vi "WaveGraphView.vi"() -> ()   [LabVIEW 2014]
uses:
  GlobalData/GlobalData.vi
panel:
  in  "btnInitial":bool
  in  "太線(+3)":bool
  in  "自動スケール":bool
  in  "軸本数":u16(ring)=4 items=["２"=2, "４"=4, "６"=6, "８"=8]
  in  "MIN":dbl format="%#_6f"
  in  "MAX":dbl format="%#_6f"
  in  "Y軸":u16(ring) items=["No.", "時間HH:MM:SS.S", "M1回転rpm", "M2回転rpm", "M3回転rpm", "M1トルクN･m", "M2トルクN･m", "M3トルクN･m"]
  in  "プロットCH":u16(ring) items=["No.", "時間HH:MM:SS.S", "M1回転rpm", "M2回転rpm", "M3回転rpm", "M1トルクN･m", "M2トルクN･m", "M3トルクN･m", "", "", "", "", "", "", "", "", "", "", "供試体温度1℃", "供試体温度2℃", "供試体温度3℃", "動力盤温度℃", "軸受温度1℃", "軸受温度2℃", "軸受温度3℃", "", "効率"]
  in  "名称":string
  in  "色":u32(colorbox)
  in  "btnAddCursor":bool
  in  "btnScaleLegendVis":bool
  in  "btnLegVis":bool
  in  "btnCursorLegendVis":bool
  out "波形グラフ":waveform(dbl)[](graph)
  # "表示"
  # "カーソル"
  # "グラフCH設定"
  # "右クリック→カーソルを作成→複数プロット。さらに右クリック→監視→全てのプロット"
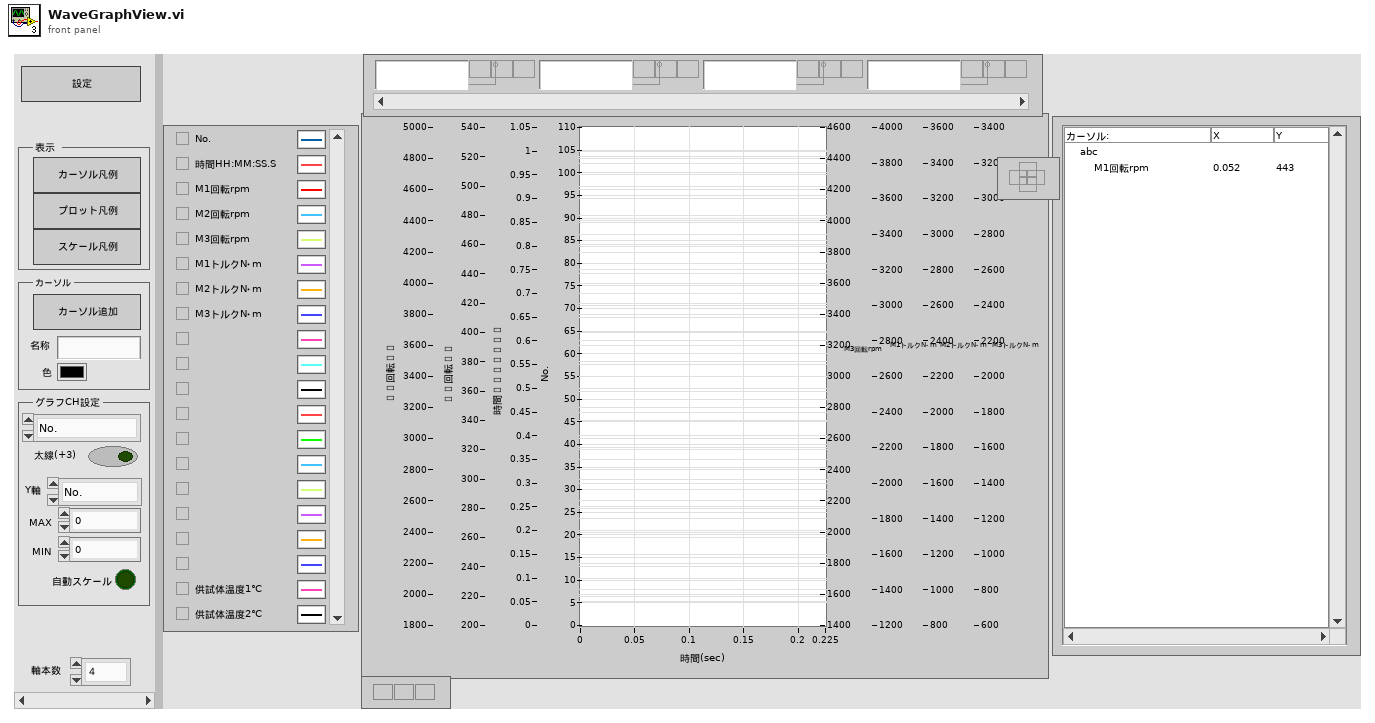
[diagram p1: front panel]
types:
  T1 = typedef "eventvkey.ctl" = enum16{"ASCII", "Enter", "Return", "Shift", "Ctrl", "Alt", "Cmd", "Opt", "Caps", "NumLock", "Clear", "Break", "Up", "Down", "Left", "Right", "Insert", "Delete", "Home", "End", "PageUp", "PageDown", "Escape", "Help", "Pause", "ScrollLock", "F1", "F2", "F3", "F4", "F5", "F6", "F7", "F8", "F9", "F10", "F11", "F12", "F13", "F14", "F15", "F16", "F17", "F18", "F19", "F20", "F21", "F22", "F23", "F24", "Play", "VolumeUp", "VolumeDown", "Mute", "Two Byte Char"}
  T2 = typedef "LVRangeTypeDef.ctl" = cluster{"Minimum":dbl, "Maximum":dbl, "Increment":dbl, "Minor Increment":dbl, "Start":dbl}
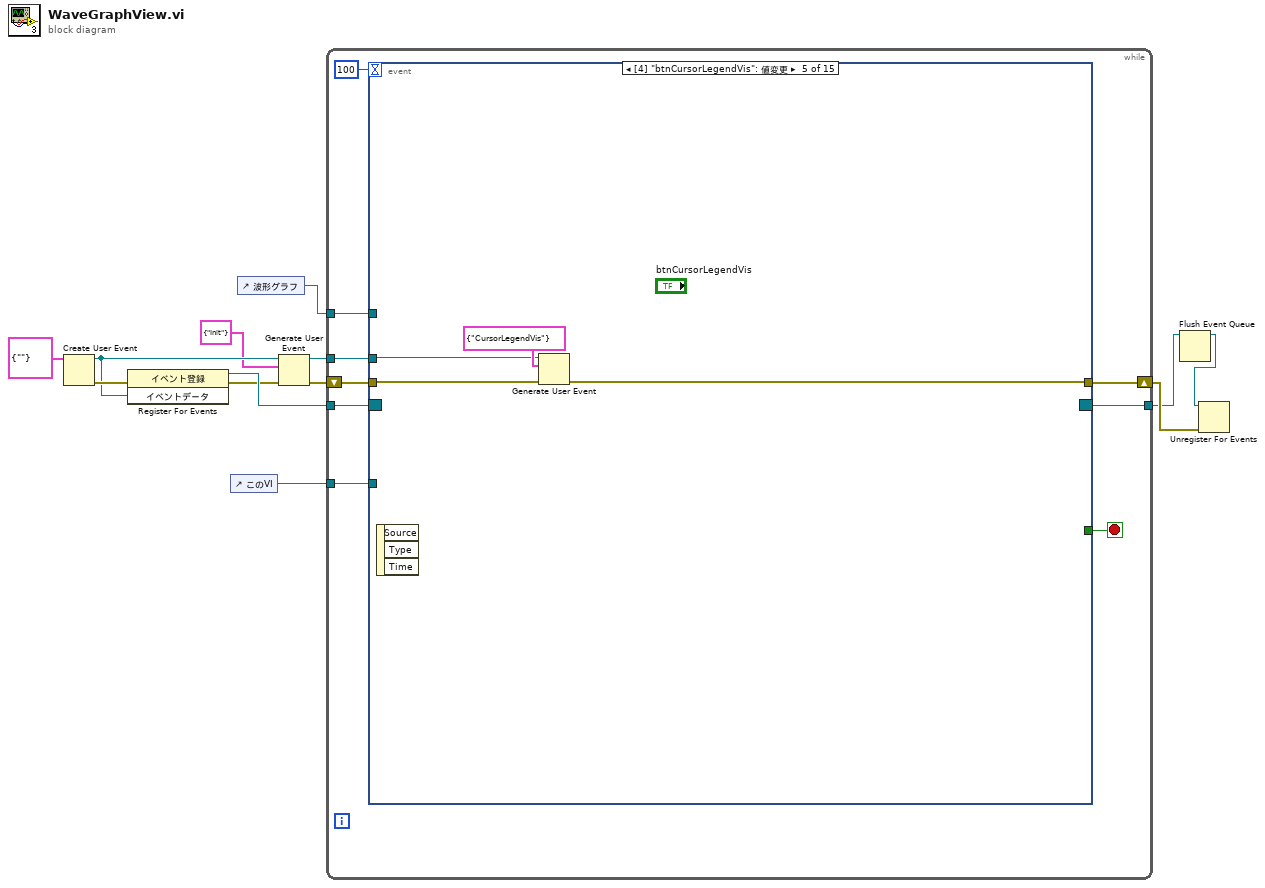
[diagram p0: block diagram]
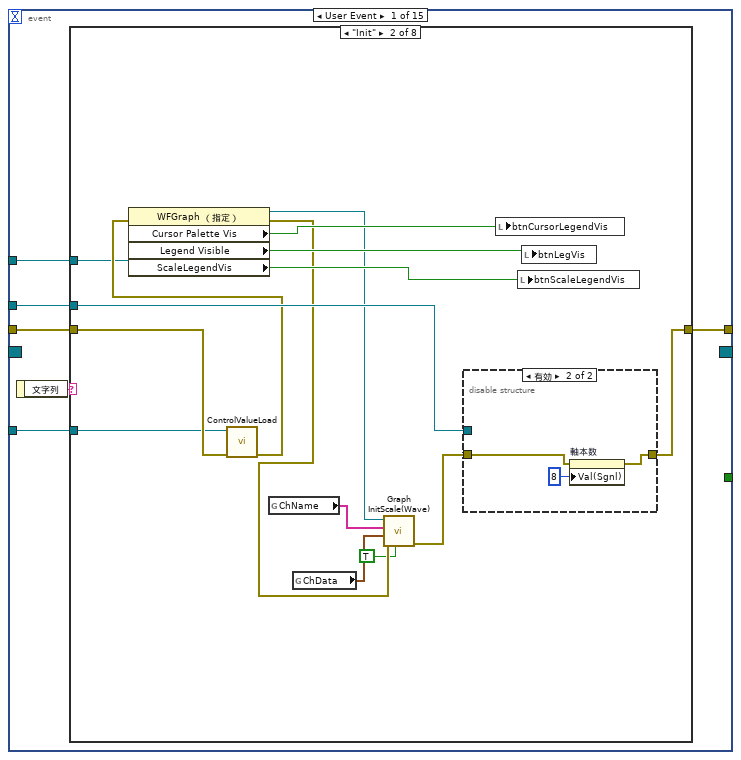
[diagram p2: hidden frame]
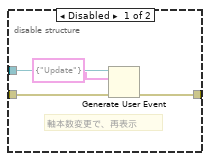
[diagram p4: hidden frame]
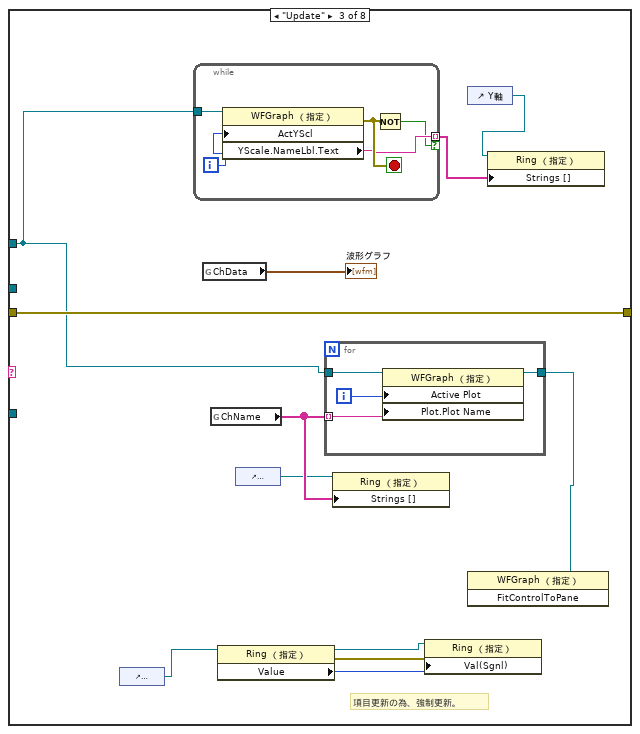
[diagram p5: hidden frame]
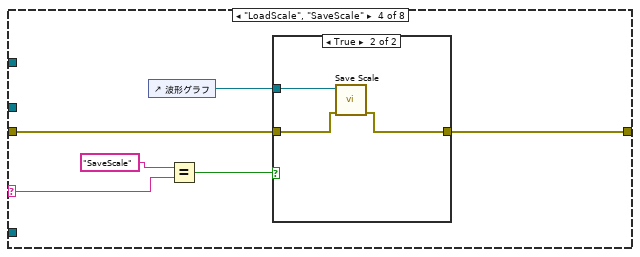
[diagram p6: hidden frame]
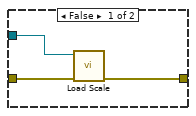
[diagram p7: hidden frame]
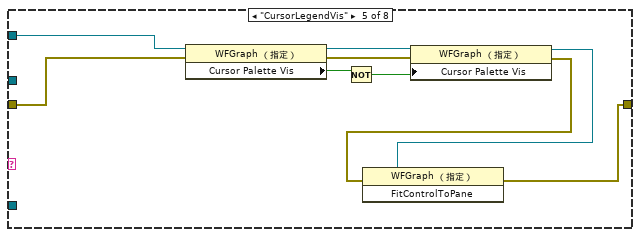
[diagram p8: hidden frame]
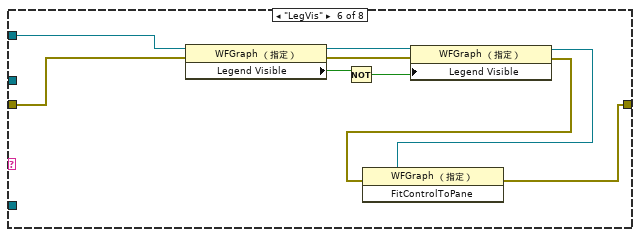
[diagram p9: hidden frame]
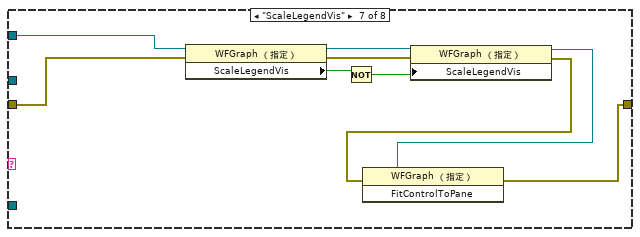
[diagram p10: hidden frame]
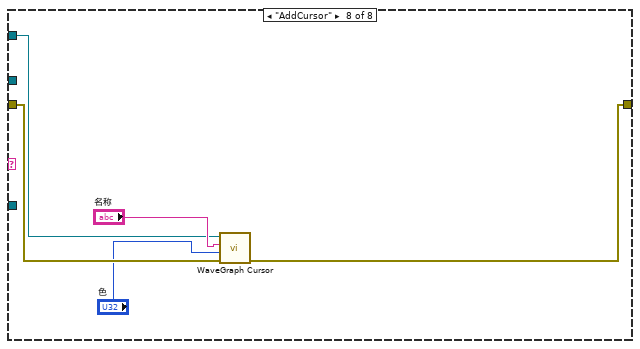
[diagram p11: hidden frame]
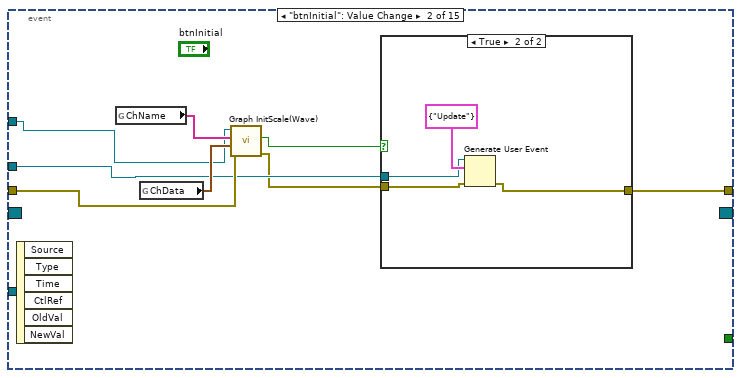
[diagram p12: hidden frame]
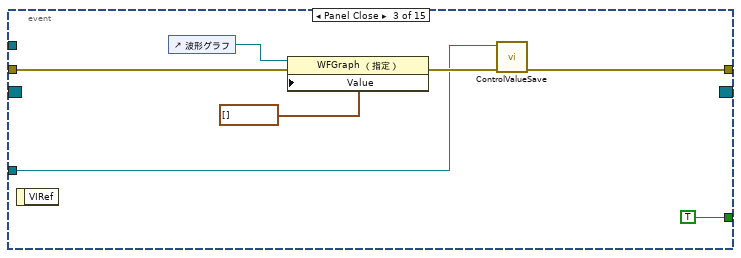
[diagram p14: hidden frame]
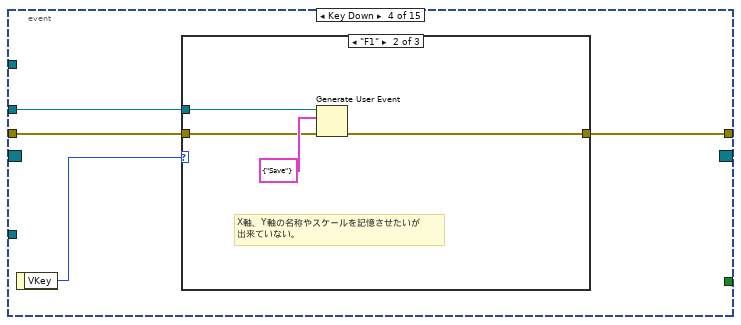
[diagram p15: hidden frame]
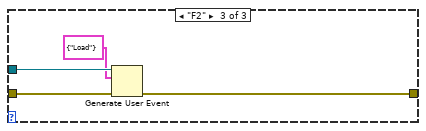
[diagram p17: hidden frame]
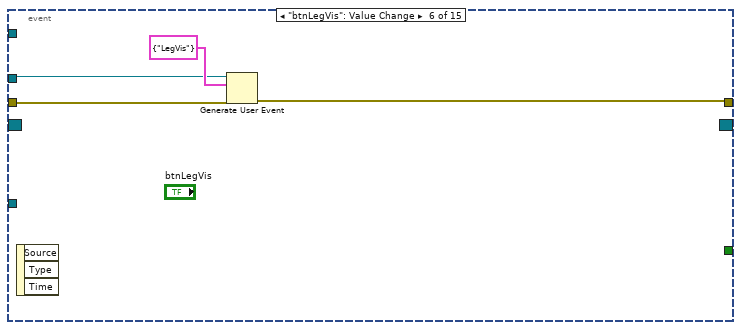
[diagram p18: hidden frame]
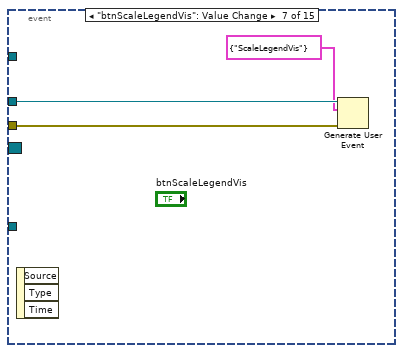
[diagram p19: hidden frame]
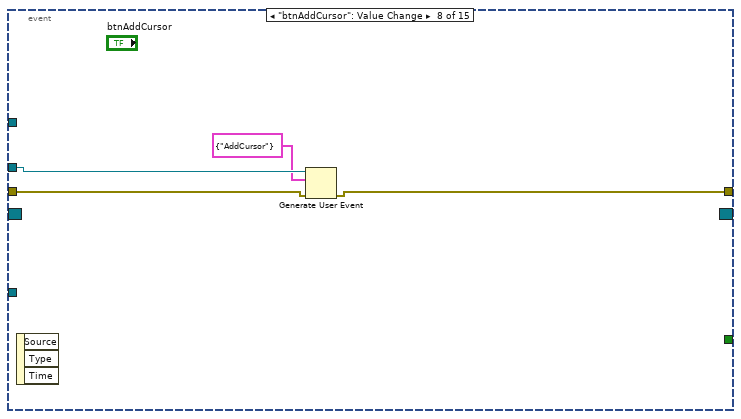
[diagram p20: hidden frame]
diagram:
  n1 = Create User Event(user event datatype=cluster{"文字列":string} {"文字列"=""} ("イベントデータ")) -> (user event=w10:refnum<user-event>, error out=w11:errorcluster)  [unwired: 1 in]
  n2 = register-events(error in=w11, w10) -> (reference out=w13:refnum<event-registration>, error out=w9:errorcluster)  [unwired: 1 in]
  n3 = control-ref of="このVI"() -> (w5:refnum<vi>)
  n4 = control-ref of="波形グラフ"() -> (w3:refnum<vi>)
  n5 = Generate User Event(user event=w10, event data cluster=cluster{"文字列":string} {"文字列"="Init"} ("イベントデータ"), error in=w9) -> (user event out=w6:refnum<user-event>, error out=w8:errorcluster)  [unwired: 1 in]
  n6 = while {
    tunnel: w13 -> [w21]
    tunnel: [w20] -> w2
    tunnel: w6 -> [w19]
    tunnel: w5 -> [w18]
    shift-right: [w16] -> w4
    shift-left: w8 -> [w17]
    tunnel: w3 -> [w15]
    stop <- w22 stop-if-true
    n7 = event shown="[4] \"btnCursorLegendVis\": 値変更" {
      selector: w21 -> [_ _ _ _ _ _ _ _ _ _ _ _ _ _ _]
      dyn-events: [_ _ _ _ _ _ _ _ _ _ _ _ _ _ _] -> w20
      timeout: 100 -> [_ _ _ _ _ _ _ _ _ _ _ _ _ _ _]
      tunnel: [_ _ TRUE _ _ _ _ _ _ _ _ _ _ _ _] -> w22
      tunnel: w19 -> [w27 w120 _ w139 w151 w156 w160 w164 _ _ _ _ w206 _ _]
      tunnel: w18 -> [w26 _ w132 _ _ _ _ _ _ _ _ _ _ _ _]
      tunnel: w17 -> [w25 w121 w134 w138 w153 w155 w158 w162 w169 _ w194 _ w205 _ w238]
      tunnel: [w24 w118 w131 w137 w150 w154 _ w161 w168 _ w187 _ w203 _ w237] -> w16
      tunnel: w15 -> [w23 w117 _ _ _ _ _ _ w171 w184 w186 w202 w209 w223 _]
      event User Event {
        n8 = event-data() -> ("文字列"=w28:string)  [unwired: 1 in]
        n9 = case shown="\"Init\"" w28 {
          selector: w28 -> [_ _ _ w74 _ _ _ _]
          tunnel: w27 -> [_ w42 _ _ _ _ _ _]
          tunnel: w26 -> [_ w41 _ _ _ _ _ _]
          tunnel: w25 -> [w29 w44 w62 w77 w89 w98 w107 w116]
          tunnel: [w29 w43 w62 w76 w86 w95 w104 w115] -> w24
          tunnel: w23 -> [_ w36 w52 _ w85 w94 w103 w112]
          frame Default {
          }
          frame "Init" {
            n10 = call "ControlValueLoad.vi"("err(in)"=w44, "VI refnum"=w41) -> ("err(out)"=w37:errorcluster)  [unwired: 9 in]
            n11 = property class="WFGraph （指定）"(reference=w36, error in=w37) -> (reference out=w30:refnum<vi>, error out=w33:errorcluster, "Cursor Palette Vis"=w40:bool, "Legend Visible"=w39:bool, "ScaleLegendVis"=w38:bool)
            n12 = global read "GlobalData.vi" "ChName"() -> (w35:string[])
            n13 = global read "GlobalData.vi" "ChData"() -> (w34:waveform(dbl)[])
            n14 = call "Graph InitScale(Wave).vi"("初回?"=TRUE, "error in (no error)"=w33, "ChData"=w34, "ChName"=w35, "波形グラフ(ref)"=w30) -> ("error out"=w32:errorcluster)  [unwired: 5 in, 1 out]
            n15 = disable-structure shown="有効" {
              disable-tunnel: [w48 w51] -> w43
              disable-tunnel: w42 -> [w47 _]
              disable-tunnel: w32 -> [w45 w50]
              frame Disabled {
                # "軸本数変更で、再表示"
                n16 = Generate User Event(user event=w47, event data cluster=cluster{"文字列":string} {"文字列"="Update"} ("イベントデータ"), error in=w45) -> (error out=w48:errorcluster)  [unwired: 1 in, 1 out]
              }
              frame Enabled {
                n17 = property on="軸本数" class="Ring （指定）"(error in=w50, "Val(Sgnl)"=u16 8 ("値（信号）")) -> (error out=w51:errorcluster)  [unwired: 1 in, 1 out]
              }
            }
            n18 = local write "btnCursorLegendVis"(w40) -> ()
            n19 = local write "btnScaleLegendVis"(w38) -> ()
            n20 = local write "btnLegVis"(w39) -> ()
          }
          frame "Update" {
            # "項目更新の為、強制更新。"
            n21 = control-ref of="プロットCH"() -> (w53:refnum<vi>)
            n22 = while {
              tunnel: w52 -> [w68]
              tunnel: [w65] -> w58 mode=indexing if=w64
              i -> [w67]
              stop <- w66 stop-if-true
              n23 = property class="WFGraph （指定）"(reference=w68, "ActYScl"=w67) -> (error out=w66:errorcluster, "YScale.NameLbl.Text"=w65:string)  [unwired: 1 in, 1 out]
              n24 = Not(x=w66) -> (.not. x?=w64:bool)
            }
            n25 = global read "GlobalData.vi" "ChData"() -> (→"波形グラフ":waveform(dbl)[])
            n26 = global read "GlobalData.vi" "ChName"() -> (w61:string[])
            n27 = property on="プロパティノード" class="Ring （指定）"(reference=w53) -> (reference out=w54:refnum<vi>, error out=w56:errorcluster, "Value"=w55:u16)  [unwired: 1 in]
            n28 = control-ref of="プロットCH"() -> (w60:refnum<vi>)
            n29 = for {
              tunnel: w52 -> [w72]
              tunnel: w61 -> [w71] mode=indexing
              tunnel: [w69] -> w57
              i -> [w70]
              n30 = property class="WFGraph （指定）"(reference=w72, "Active Plot"=w70, "Plot.Plot Name"=w71) -> (reference out=w69:refnum<vi>)  [unwired: 1 in, 1 out]
            }
            n31 = property class="Ring （指定）"(reference=w60, "Strings []"=w61) -> ()  [unwired: 1 in, 2 out]
            n32 = property on="プロパティノード" class="Ring （指定）"(reference=w54, error in=w56, "Val(Sgnl)"=w55) -> ()  [unwired: 2 out]
            n33 = control-ref of="Y軸"() -> (w59:refnum<vi>)
            n34 = invoke class="WFGraph （指定）" method="FitControlToPane"(reference=w57) -> ()  [unwired: 2 in, 3 out]
            n35 = property class="Ring （指定）"(reference=w59, "Strings []"=w58) -> ()  [unwired: 1 in, 2 out]
          }
          frame "LoadScale", "SaveScale" {
            n36 = control-ref of="波形グラフ"() -> (w78:refnum<vi>)
            n37 = Equal?(x="SaveScale", y=w74) -> (x = y?=w73:bool)
            n38 = case shown="TRUE" w73 {
              tunnel: w78 -> [w81 w84]
              tunnel: w77 -> [w80 w83]
              tunnel: [w79 w82] -> w76
              frame False {
                n39 = call "Load Scale.vi"("err in"=w80, "WaveformGraph入力"=w81) -> ("err out"=w79:errorcluster)  [unwired: 9 in]
              }
              frame True {
                n40 = call "Save Scale.vi"("err in"=w83, "WaveformGraph入力"=w84) -> ("error out"=w82:errorcluster)  [unwired: 9 in]
              }
            }
          }
          frame "CursorLegendVis" {
            n41 = property class="WFGraph （指定）"(reference=w85, error in=w89) -> (reference out=w90:refnum<vi>, error out=w91:errorcluster, "Cursor Palette Vis"=w93:bool)
            n42 = Not(x=w93) -> (.not. x?=w92:bool)
            n43 = property class="WFGraph （指定）"(reference=w90, error in=w91, "Cursor Palette Vis"=w92) -> (reference out=w88:refnum<vi>, error out=w87:errorcluster)
            n44 = invoke class="WFGraph （指定）" method="FitControlToPane"(reference=w88, error in=w87) -> (error out=w86:errorcluster)  [unwired: 1 in, 2 out]
          }
          frame "LegVis" {
            n45 = property class="WFGraph （指定）"(reference=w94, error in=w98) -> (reference out=w99:refnum<vi>, error out=w100:errorcluster, "Legend Visible"=w102:bool)
            n46 = Not(x=w102) -> (.not. x?=w101:bool)
            n47 = property class="WFGraph （指定）"(reference=w99, error in=w100, "Legend Visible"=w101) -> (reference out=w97:refnum<vi>, error out=w96:errorcluster)
            n48 = invoke class="WFGraph （指定）" method="FitControlToPane"(reference=w97, error in=w96) -> (error out=w95:errorcluster)  [unwired: 1 in, 2 out]
          }
          frame "ScaleLegendVis" {
            n49 = property class="WFGraph （指定）"(reference=w103, error in=w107) -> (reference out=w108:refnum<vi>, error out=w109:errorcluster, "ScaleLegendVis"=w111:bool)
            n50 = Not(x=w111) -> (.not. x?=w110:bool)
            n51 = property class="WFGraph （指定）"(reference=w108, error in=w109, "ScaleLegendVis"=w110) -> (reference out=w106:refnum<vi>, error out=w105:errorcluster)
            n52 = invoke class="WFGraph （指定）" method="FitControlToPane"(reference=w106, error in=w105) -> (error out=w104:errorcluster)  [unwired: 1 in, 2 out]
          }
          frame "AddCursor" {
            n53 = call "WaveGraph Cursor.vi"("エラー入力（エラーなし）"=w116, "色"="色", "名称"="名称", "WaveformGraph入力"=w112) -> ("エラー出力"=w115:errorcluster)  [unwired: 7 in]
          }
        }
      }
      event "btnInitial": Value Change {
        n54 = event-data() -> ()  [unwired: 1 in, 6 out]
        n55 = global read "GlobalData.vi" "ChName"() -> (w124:string[])
        n56 = global read "GlobalData.vi" "ChData"() -> (w123:waveform(dbl)[])
        n57 = call "Graph InitScale(Wave).vi"("error in (no error)"=w121, "ChData"=w123, "ChName"=w124, "波形グラフ(ref)"=w117) -> ("error out"=w119:errorcluster, "OK"=w122:bool)  [unwired: 6 in]
        n58 = case shown="TRUE" w122 {
          tunnel: w120 -> [_ w128]
          tunnel: w119 -> [w125 w127]
          tunnel: [w125 w126] -> w118
          frame False {
          }
          frame True {
            n59 = Generate User Event(user event=w128, event data cluster=cluster{"文字列":string} {"文字列"="Update"} ("イベントデータ"), error in=w127) -> (error out=w126:errorcluster)  [unwired: 1 in, 1 out]
          }
        }
      }
      event Panel Close {
        n60 = event-data() -> ()  [unwired: 1 in, 1 out]
        n61 = control-ref of="波形グラフ"() -> (w130:refnum<vi>)
        n62 = property class="WFGraph （指定）"(reference=w130, error in=w134, "Value"=waveform(dbl)[] [] ("値")) -> (error out=w133:errorcluster)  [unwired: 1 out]
        n63 = call "ControlValueSave.vi"("err(in)"=w133, "VI refnum"=w132) -> ("err(out)"=w131:errorcluster)  [unwired: 9 in]
      }
      event Key Down {
        n64 = event-data() -> ("VKey"=w140:T1)  [unwired: 1 in]
        n65 = case shown="\"F1\"" w140 {
          tunnel: w139 -> [_ w145 w149]
          tunnel: w138 -> [w141 w143 w147]
          tunnel: [w141 w142 w146] -> w137
          frame "ASCII", Default {
          }
          frame "F1" {
            # "X軸、Y軸の名称やスケールを記憶させたいが\n出来ていない。"
            n66 = Generate User Event(user event=w145, event data cluster=cluster{"文字列":string} {"文字列"="Save"} ("イベントデータ"), error in=w143) -> (error out=w142:errorcluster)  [unwired: 1 in, 1 out]
          }
          frame "F2" {
            n67 = Generate User Event(user event=w149, event data cluster=cluster{"文字列":string} {"文字列"="Load"} ("イベントデータ"), error in=w147) -> (error out=w146:errorcluster)  [unwired: 1 in, 1 out]
          }
        }
      }
      event "btnCursorLegendVis": Value Change {
        n68 = event-data() -> ()  [unwired: 1 in, 3 out]
        n69 = Generate User Event(user event=w151, event data cluster=cluster{"文字列":string} {"文字列"="CursorLegendVis"} ("イベントデータ"), error in=w153) -> (error out=w150:errorcluster)  [unwired: 1 in, 1 out]
      }
      event "btnLegVis": Value Change {
        n70 = event-data() -> ()  [unwired: 1 in, 3 out]
        n71 = Generate User Event(user event=w156, event data cluster=cluster{"文字列":string} {"文字列"="LegVis"} ("イベントデータ"), error in=w155) -> (error out=w154:errorcluster)  [unwired: 1 in, 1 out]
      }
      event "btnScaleLegendVis": Value Change {
        n72 = event-data() -> ()  [unwired: 1 in, 3 out]
        n73 = Generate User Event(user event=w160, event data cluster=cluster{"文字列":string} {"文字列"="ScaleLegendVis"} ("イベントデータ"), error in=w158) -> ()  [unwired: 1 in, 2 out]
      }
      event "btnAddCursor": Value Change {
        n74 = event-data() -> ()  [unwired: 1 in, 3 out]
        n75 = Generate User Event(user event=w164, event data cluster=cluster{"文字列":string} {"文字列"="AddCursor"} ("イベントデータ"), error in=w162) -> (error out=w161:errorcluster)  [unwired: 1 in, 1 out]
      }
      event "プロットCH": Value Change {
        n76 = event-data() -> ()  [unwired: 1 in, 1 out]
        n77 = property class="WFGraph （指定）"(reference=w171, error in=w169, "Active Plot"="プロットCH") -> (reference out=w167:refnum<vi>, error out=w168:errorcluster, "Plot.YScaleIdx"=w166:u32)
        n78 = property class="WFGraph （指定）"(reference=w167, "ActYScl"=w166) -> ("YScale.Range"=w165:T2)  [unwired: 1 in, 2 out]
        n79 = To Unsigned Word Integer(number=w166) -> (unsigned 16bit integer=w174:u16)
        n80 = local write "Y軸"(w174) -> ()
        n81 = Unbundle By Name(w165) -> ("Maximum"=w173:dbl, "Minimum"=w172:dbl)
        n82 = local write "MIN"(w172) -> ()
        n83 = local write "MAX"(w173) -> ()
      }
      event "Y軸": Value Change {
        n84 = event-data() -> ()  [unwired: 1 in, 6 out]
        n85 = local read "プロットCH"() -> (w183:u16)
        n86 = property class="WFGraph （指定）"(reference=w184, "Active Plot"=w183) -> (reference out=w177:refnum<vi>, error out=w181:errorcluster, "Plot"=w182:refnum<vi>)  [unwired: 1 in]
        n87 = property class="Plot"(reference=w182, error in=w181, "YScaleIdx"="Y軸") -> (error out=w175:errorcluster)  [unwired: 1 out]
        n88 = property class="WFGraph （指定）"(reference=w177, error in=w175, "ActYScl"="Y軸") -> ("YScale.Range"=w180:T2)  [unwired: 2 out]
        n89 = Unbundle By Name(w180) -> ("Maximum"=w179:dbl, "Minimum"=w178:dbl)
        n90 = local write "MAX"(w179) -> ()
        n91 = local write "MIN"(w178) -> ()
      }
      event "MAX", "MIN": Value Change {
        n92 = event-data() -> ()  [unwired: 1 in, 6 out]
        n93 = local read "Y軸"() -> (w185:u16)
        n94 = property class="WFGraph （指定）"(reference=w186, error in=w194, "ActYScl"=w185) -> (reference out=w192:refnum<vi>, error out=w190:errorcluster, "YScale.Range"=w193:T2)
        n95 = Bundle By Name(cluster=w193, "Maximum"="MAX", "Minimum"="MIN") -> (w191:T2)
        n96 = property class="WFGraph （指定）"(reference=w192, error in=w190, "YScale.Range"=w191) -> (error out=w187:errorcluster)  [unwired: 1 out]
      }
      event "自動スケール": Value Change {
        n97 = event-data() -> ()  [unwired: 1 in, 6 out]
        n98 = local read "Y軸"() -> (w201:u16)
        n99 = property class="WFGraph （指定）"(reference=w202, "ActYScl"=w201, "YScale.ScaleFit"=u8 1 ("Yスケール.スケールフィット")) -> (reference out=w199:refnum<vi>, error out=w198:errorcluster)  [unwired: 1 in]
        n100 = property class="WFGraph （指定）"(reference=w199, error in=w198) -> ("YScale.Range"=w197:T2)  [unwired: 2 out]
        n101 = Unbundle By Name(w197) -> ("Maximum"=w196:dbl, "Minimum"=w195:dbl)
        n102 = local write "MAX"(w196) -> ()
        n103 = local write "MIN"(w195) -> ()
      }
      event "軸本数": Value Change {
        n104 = event-data() -> ()  [unwired: 1 in, 6 out]
        n105 = while {
          tunnel: w209 -> [w217]
          tunnel: [w211] -> w208
          tunnel: w205 -> [w210]
          i -> [w216]
          stop <- w212 stop-if-true
          n106 = To Unsigned Word Integer(number=w216) -> (unsigned 16bit integer=w213:u16)
          n107 = Less?(x=w213, y="軸本数") -> (x < y?=w214:bool)
          n108 = property class="WFGraph （指定）"(reference=w217, error in=w210, "ActYScl"=w216, "YScale.Visible"=w214) -> (reference out=w211:refnum<vi>, error out=w212:errorcluster)
        }
        n109 = invoke class="WFGraph （指定）" method="FitControlToPane"(reference=w208) -> (error out=w204:errorcluster)  [unwired: 2 in, 2 out]
        n110 = Generate User Event(user event=w206, event data cluster=cluster{"文字列":string} {"文字列"="Update"} ("イベントデータ"), error in=w204) -> (error out=w203:errorcluster)  [unwired: 1 in, 1 out]
      }
      event Timeout {
        n111 = event-data() -> ()  [unwired: 1 in, 3 out]
        n112 = local read "プロットCH"() -> (w222:u16)
        n113 = feedback-in #1("太線(+3)") -> ()
        n114 = feedback #1() -> (w226:bool)  [unwired: 1 in]
        n115 = Build Array("太線(+3)", w226) -> (w225:bool[])
        n116 = property class="WFGraph （指定）"(reference=w223, "Active Plot"=w222) -> (reference out=w220:refnum<vi>, "Plot.Line Width"=w221:u8)  [unwired: 1 in, 1 out]
        n117 = Boolean Array To Number(Boolean array=w225) -> (number=w224:u32)
        n118 = case shown="1" w224 {
          tunnel: w221 -> [_ w229 w234]
          tunnel: w220 -> [_ w231 w236]
          tunnel: 3 -> [_ w228 w233]
          frame 0, Default {
          }
          frame 2 {
            # "ON->OFF"
            n119 = Subtract(x=w229, y=w228) -> (x-y=w227:i32)
            n120 = To Unsigned Byte Integer(number=w227) -> (unsigned 8bit integer=w230:u8)
            n121 = property class="WFGraph （指定）"(reference=w231, "Plot.Line Width"=w230) -> ()  [unwired: 1 in, 2 out]
          }
          frame 1 {
            # "OFF->ON"
            n122 = Add(x=w234, y=w233) -> (x+y=w232:i32)
            n123 = To Unsigned Byte Integer(number=w232) -> (unsigned 8bit integer=w235:u8)
            n124 = property class="WFGraph （指定）"(reference=w236, "Plot.Line Width"=w235) -> ()  [unwired: 1 in, 2 out]
          }
        }
      }
      event "波形グラフ": Plot Attribute Change {
        n125 = event-data() -> ("PlotIdx"=w239:i32)  [unwired: 1 in, 7 out]
        n126 = property on="プロットCH" class="Ring （指定）"(error in=w238, "Val(Sgnl)"=w239) -> (error out=w237:errorcluster)  [unwired: 1 in, 1 out]
      }
    }
  }
  n127 = Flush Event Queue(0:w2) -> (8:w1:refnum<event-registration>)  [unwired: 5 in, 2 out]
  n128 = Unregister For Events(event registration refnum=w1, error in=w4) -> ()  [unwired: 1 out]
